vi "Test_CreateTable.vi"() -> ()   [LabVIEW 2020]
uses:
  C:/Program Files (x86)/National Instruments/LabVIEW 2018/vi.lib/Viviota/Viviota ORM/libraries/kdb/KpNet.KdbPlusClient.dll
  Program Files (x86)/National Instruments/LabVIEW 2018/vi.lib/Viviota/Viviota ORM/libraries/kdb/KpNet.KdbPlusClient.dll
  System.Data
  <vilib>/Viviota/VIV_Tools/Helpers.lvlib
panel:
  out "error out 3":errorcluster
  out "Array 7":string[](array[string])
  out "Array 6":variant[](array[variant])
  out "error out 2":errorcluster
  out "FieldCount 2":i32
  out "variant 4":variant
  out "variant 3":variant
  out "Array 5":string[](array[string])
  out "Array 4":variant[](array[variant])
  out "variant":variant
  out "GetName":string
  out "FieldCount":i32
  out "error out":errorcluster
  out "Array 3":string[](array[string])
  out "Array 2":variant[](array[variant])
  out "Read":bool
  out "Array":string[](array[string])
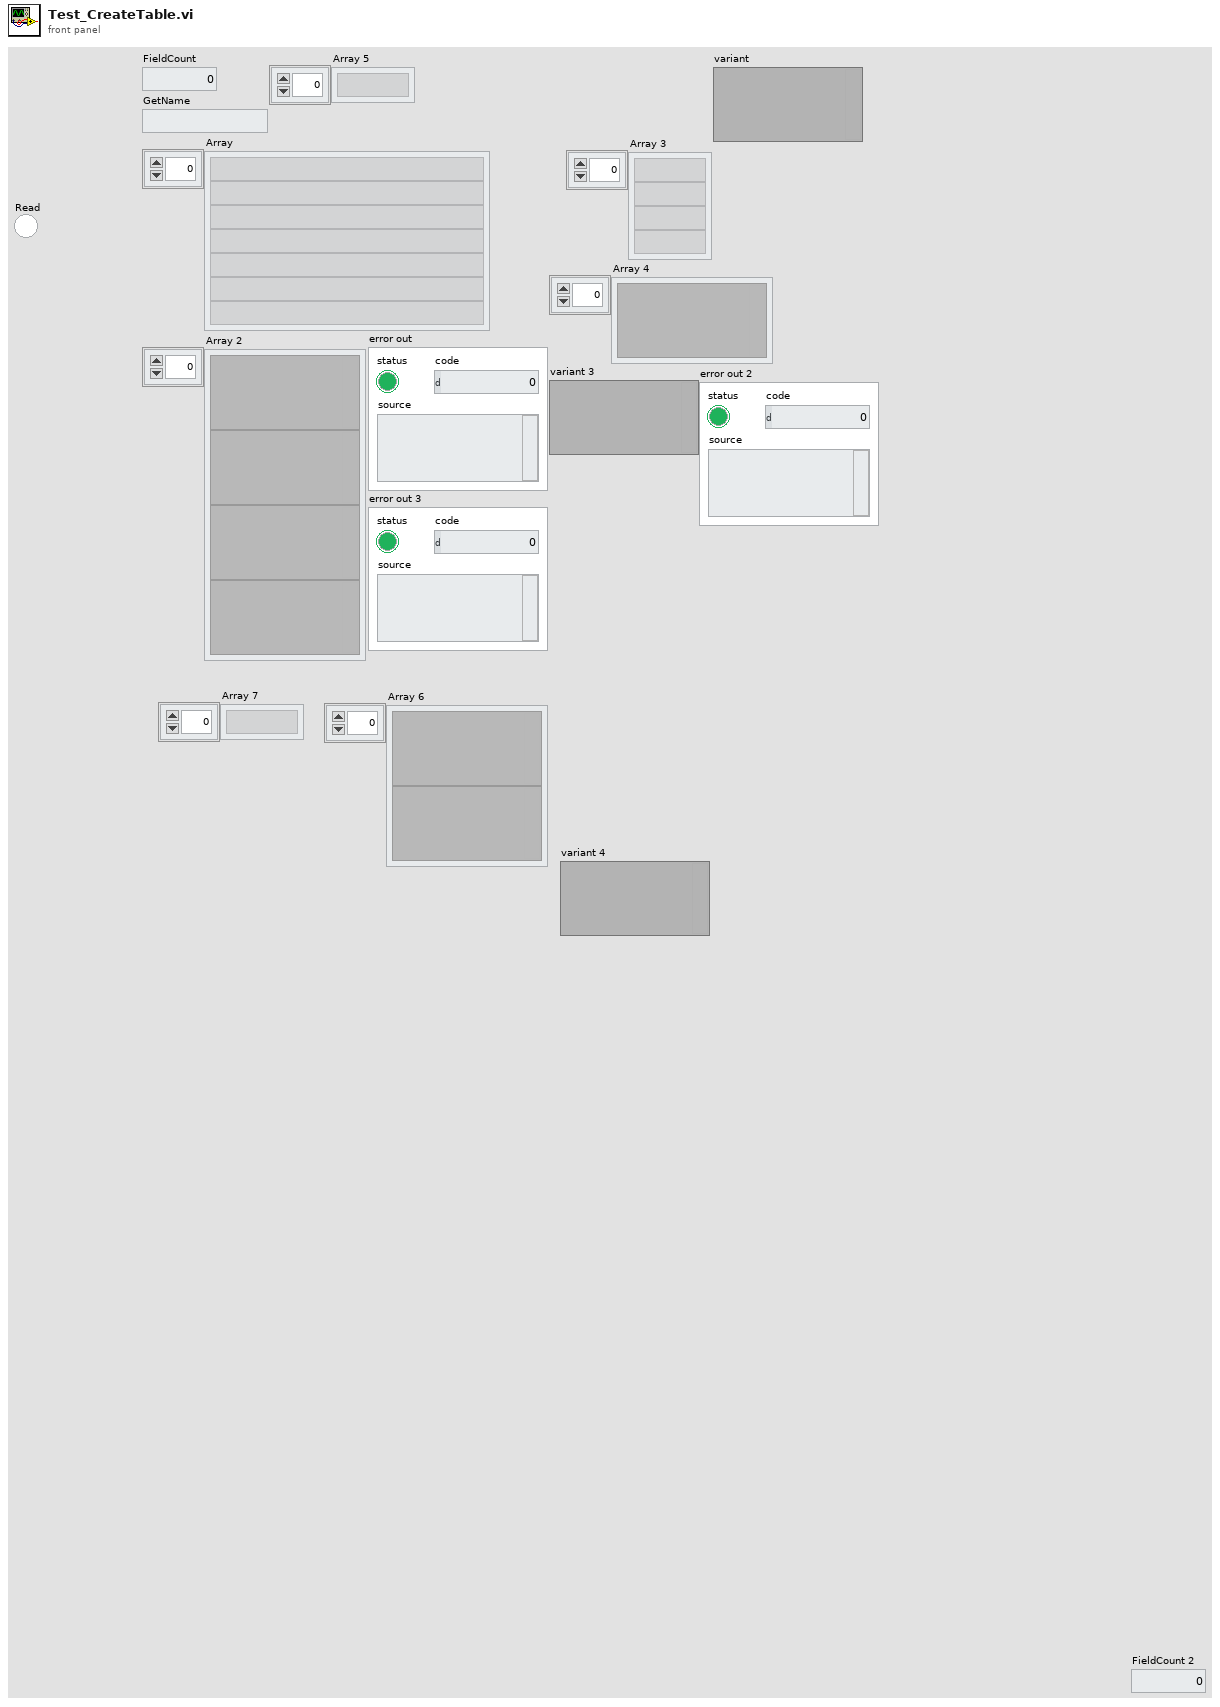
[diagram p1: front panel]
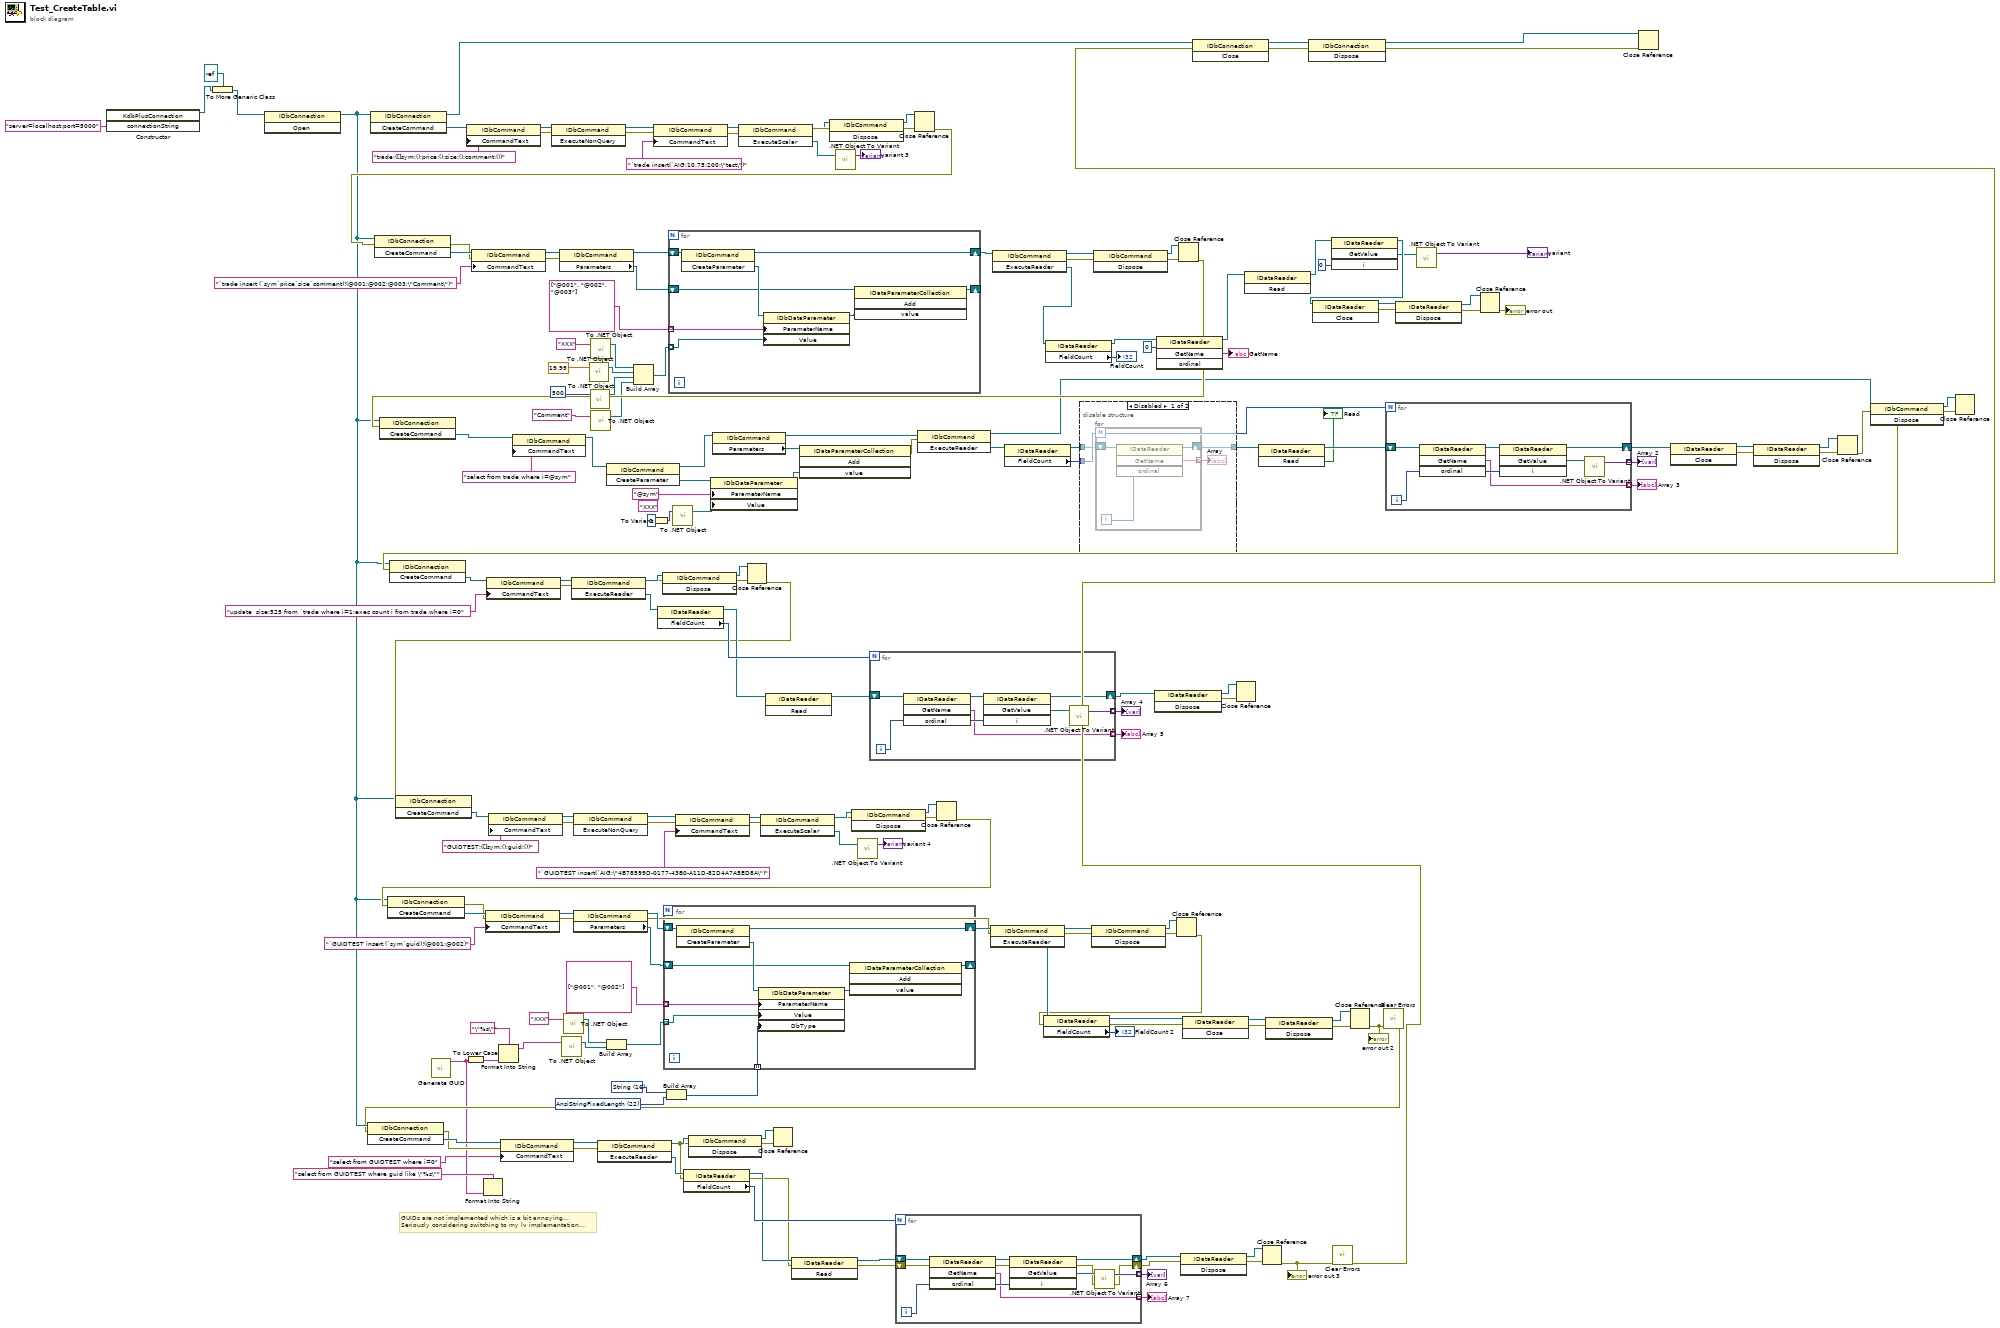
[diagram p0: block diagram]
diagram:
  w32 = 22 items=["AnsiString"=0, "Binary"=1, "Byte"=2, "Boolean"=3, "Currency"=4, "Date"=5, "DateTime"=6, "Decimal"=7, "Double"=8, "Guid"=9, "Int16"=10, "Int32"=11, "Int64"=12, "Object"=13, "SByte"=14, "Single"=15, "String"=16, "Time"=17, "UInt16"=18, "UInt32"=19, "UInt64"=20, "VarNumeric"=21, "AnsiStringFixedLength"=22, "StringFixedLength"=23, "Xml"=25, "DateTime2"=26, "DateTimeOffset"=27] ("DbType")
  w33 = 16 items=["AnsiString"=0, "Binary"=1, "Byte"=2, "Boolean"=3, "Currency"=4, "Date"=5, "DateTime"=6, "Decimal"=7, "Double"=8, "Guid"=9, "Int16"=10, "Int32"=11, "Int64"=12, "Object"=13, "SByte"=14, "Single"=15, "String"=16, "Time"=17, "UInt16"=18, "UInt32"=19, "UInt64"=20, "VarNumeric"=21, "AnsiStringFixedLength"=22, "StringFixedLength"=23, "Xml"=25, "DateTime2"=26, "DateTimeOffset"=27] ("DbType")
  (unwired) "XXX"
  # "GUIDs are not implemented which is a bit annoying...\nSeriously considering switching to my lv implementation..."
  n1 = constructor class="KdbPlusConnection"("connectionString"="server=localhost;port=5000") -> (reference out=w123:refnum<k24>)  [unwired: 3 in, 3 out]
  n2 = To More Generic Class(target class=refnum<k24> refnum ("connection"), reference=w123) -> (generic class reference=w122:refnum<k24>)
  n3 = invoke class="IDbConnection" method="Open"(reference=w122) -> (reference out=w25:refnum<k24>)  [unwired: 2 in, 2 out]
  n4 = invoke class="IDbConnection" method="CreateCommand"(reference=w25) -> (reference out=w125:refnum<k24>, "CreateCommand"=w189:refnum<k24>)  [unwired: 2 in, 1 out]
  n5 = call <vilib>:"Generate GUID.vi"() -> ("GUID"=w2:string)  [unwired: 9 in, 2 out]
  n6 = To Lower Case(string=w2) -> (all lower case string=w26:string)
  n7 = property class="IDbCommand"(reference=w189, "CommandText"="trade:([]sym:();price:();size:();comment:())") -> (reference out=w187:refnum<k24>, error out=w172:errorcluster)  [unwired: 1 in]
  n8 = Format Into String(format string="select from GUIDTEST where guid like \"%s\"" ("CommandText"), w2) -> ()  [unwired: 2 in, 2 out]
  n9 = Format Into String(format string="\"%s\"", w26) -> (resulting string=w30:string)  [unwired: 2 in, 1 out]
  n10 = invoke class="IDbCommand" method="ExecuteNonQuery"(reference=w187, error in=w172) -> (reference out=w174:refnum<k24>, error out=w173:errorcluster)  [unwired: 1 in, 1 out]
  n11 = call <vilib>:"To .NET Object.vi"("anything"=w30) -> (".NET object"=w52:refnum<k24>)  [unwired: 1 in, 1 out]
  n12 = call <vilib>:"To .NET Object.vi"("anything"="XXX") -> (".NET object"=w53:refnum<k24>)  [unwired: 1 in, 1 out]
  n13 = call <vilib>:"To .NET Object.vi"("anything"=19.99) -> (".NET object"=w146:refnum<k24>)  [unwired: 1 in, 1 out]
  n14 = call <vilib>:"To .NET Object.vi"("anything"=500) -> (".NET object"=w145:refnum<k24>)  [unwired: 1 in, 1 out]
  n15 = call <vilib>:"To .NET Object.vi"("anything"="XXX") -> (".NET object"=w147:refnum<k24>)  [unwired: 1 in, 1 out]
  n16 = call <vilib>:"To .NET Object.vi"("anything"="Comment") -> (".NET object"=w79:refnum<k24>)  [unwired: 1 in, 1 out]
  n17 = Build Array(w53, w52) -> (w51:refnum<k24>[])
  n18 = Build Array(w147, w146, w145, w79) -> (w144:refnum<k24>[])
  n19 = To Variant(anything=0) -> (Variant=w101:variant)
  n20 = property class="IDbCommand"(reference=w174, error in=w173, "CommandText"="`trade insert(`AIG;10.75;200;\"test\")") -> (reference out=w175:refnum<k24>, error out=w170:errorcluster)
  n21 = Build Array(w33, w32) -> (w31:i32[])
  n22 = call <vilib>:"To .NET Object.vi"("anything"=w101) -> (".NET object"=w162:refnum<k24>)  [unwired: 1 in, 1 out]
  n23 = invoke class="IDbCommand" method="ExecuteScalar"(reference=w175, error in=w170) -> (reference out=w140:refnum<k24>, error out=w141:errorcluster, "ExecuteScalar"=w82:refnum<k24>)  [unwired: 1 in]
  n24 = invoke class="IDbCommand" method="Dispose"(reference=w140, error in=w141) -> (reference out=w143:refnum<k24>, error out=w142:errorcluster)  [unwired: 1 in, 1 out]
  n25 = call <vilib>:".NET Object To Variant.vi"(".NET object"=w82) -> ("variant"=→"variant 3":variant)  [unwired: 1 in, 1 out]
  n26 = Close Reference(reference=w143, error in (no error)=w142) -> (error out=w132:errorcluster)
  n27 = invoke class="IDbConnection" method="CreateCommand"(reference=w25, error in=w132) -> (error out=w134:errorcluster, "CreateCommand"=w139:refnum<k24>)  [unwired: 1 in, 1 out]
  n28 = property class="IDbCommand"(reference=w139, error in=w134, "CommandText"="`trade insert (`sym`price`size`comment)!(@001;@002;@003;\"Comment\")") -> (reference out=w154:refnum<k24>, error out=w133:errorcluster)
  n29 = property class="IDbCommand"(reference=w154, error in=w133) -> (reference out=w153:refnum<k24>, "Parameters"=w152:refnum<k24>)  [unwired: 1 out]
  n30 = for {
    tunnel: w144 -> [w198] mode=indexing
    shift-right: [w194] -> _
    shift-left: w152 -> [w195]
    shift-right: [w193] -> w151
    shift-left: w153 -> [w196]
    tunnel: string[] ["@001", "@002", "@003"] -> [w192] mode=indexing
    n31 = invoke class="IDbCommand" method="CreateParameter"(reference=w196) -> (reference out=w193:refnum<k24>, "CreateParameter"=w197:refnum<k24>)  [unwired: 2 in, 1 out]
    n32 = property class="IDbDataParameter"(reference=w197, "ParameterName"=w192, "Value"=w198) -> (reference out=w191:refnum<k24>)  [unwired: 1 in, 1 out]
    n33 = invoke class="IDataParameterCollection" method="Add"(reference=w195, "value"=w191) -> (reference out=w194:refnum<k24>)  [unwired: 2 in, 3 out]
  }
  n34 = invoke class="IDbCommand" method="ExecuteReader"(reference=w151) -> (reference out=w136:refnum<k24>, error out=w135:errorcluster, "ExecuteReader"=w113:refnum<k24>)  [unwired: 2 in]
  n35 = property class="IDataReader"(reference=w113) -> (reference out=w111:refnum<k24>, "FieldCount"=→"FieldCount":i32)  [unwired: 1 in, 1 out]
  n36 = invoke class="IDbCommand" method="Dispose"(reference=w136, error in=w135) -> (reference out=w137:refnum<k24>, error out=w138:errorcluster)  [unwired: 1 in, 1 out]
  n37 = invoke class="IDataReader" method="GetName"(reference=w111, "ordinal"=0 ("i")) -> (reference out=w108:refnum<k24>, "GetName"=→"GetName":string)  [unwired: 2 in, 2 out]
  n38 = Close Reference(reference=w137, error in (no error)=w138) -> (error out=w130:errorcluster)
  n39 = invoke class="IDbConnection" method="CreateCommand"(reference=w25, error in=w130) -> ("CreateCommand"=w131:refnum<k24>)  [unwired: 1 in, 2 out]
  n40 = property class="IDbCommand"(reference=w131, "CommandText"="select from trade where i=@sym") -> (reference out=w176:refnum<k24>)  [unwired: 1 in, 1 out]
  n41 = invoke class="IDbCommand" method="CreateParameter"(reference=w176) -> (reference out=w177:refnum<k24>, "CreateParameter"=w181:refnum<k24>)  [unwired: 2 in, 1 out]
  n42 = property class="IDbDataParameter"(reference=w181, "ParameterName"="@sym", "Value"=w162) -> (reference out=w180:refnum<k24>)  [unwired: 1 in, 1 out]
  n43 = property class="IDbCommand"(reference=w177) -> (reference out=w178:refnum<k24>, "Parameters"=w182:refnum<k24>)  [unwired: 1 in, 1 out]
  n44 = invoke class="IDataParameterCollection" method="Add"(reference=w182, "value"=w180) -> (error out=w169:errorcluster)  [unwired: 2 in, 3 out]
  n45 = invoke class="IDbCommand" method="ExecuteReader"(reference=w178, error in=w169) -> (reference out=w126:refnum<k24>, "ExecuteReader"=w164:refnum<k24>)  [unwired: 1 in, 1 out]
  n46 = property class="IDataReader"(reference=w164) -> (reference out=w161:refnum<k24>, "FieldCount"=w120:i32)  [unwired: 1 in, 1 out]
  n47 = disable-structure shown="Disabled" {
    disable-tunnel: w161 -> [w201 w207]
    disable-tunnel: [w200 w207] -> w160
    disable-tunnel: w120 -> [w199 _]
    frame Disabled {
      n48 = for {
        N: w199 -> [_]
        tunnel: [w205] -> w202 mode=indexing
        shift-right: [w206] -> w200
        shift-left: w201 -> [w204]
        i -> [w203]
        n49 = invoke class="IDataReader" method="GetName"(reference=w204, "ordinal"=w203) -> (reference out=w206:refnum<k24>, "GetName"=w205:string)  [unwired: 2 in, 2 out]
      }
      "Array" <- w202
    }
    frame Enabled {
    }
  }
  n50 = invoke class="IDataReader" method="Read"(reference=w108) -> (reference out=w107:refnum<k24>)  [unwired: 2 in, 2 out]
  n51 = invoke class="IDataReader" method="Read"(reference=w160) -> (reference out=w159:refnum<k24>, "Read"=→"Read":bool)  [unwired: 2 in, 1 out]
  n52 = invoke class="IDataReader" method="GetValue"(reference=w107, "i"=0) -> (reference out=w106:refnum<k24>, "GetValue"=w104:refnum<k24>)  [unwired: 2 in, 2 out]
  n53 = invoke class="IDataReader" method="Close"(reference=w106) -> (reference out=w115:refnum<k24>, error out=w116:errorcluster)  [unwired: 2 in, 1 out]
  n54 = for {
    N: w120 -> [_]
    shift-right: [w214] -> w158
    shift-left: w159 -> [w211]
    tunnel: [w212] -> w121 mode=indexing
    tunnel: [w208] -> w119 mode=indexing
    i -> [w209]
    n55 = invoke class="IDataReader" method="GetName"(reference=w211, "ordinal"=w209) -> (reference out=w210:refnum<k24>, "GetName"=w208:string)  [unwired: 2 in, 2 out]
    n56 = invoke class="IDataReader" method="GetValue"(reference=w210, "i"=w209) -> (reference out=w214:refnum<k24>, "GetValue"=w213:refnum<k24>)  [unwired: 2 in, 2 out]
    n57 = call <vilib>:".NET Object To Variant.vi"(".NET object"=w213) -> ("variant"=w212:variant)  [unwired: 1 in, 1 out]
  }
  "Array 2" <- w121
  "Array 3" <- w119
  n58 = invoke class="IDataReader" method="Dispose"(reference=w115, error in=w116) -> (reference out=w118:refnum<k24>, error out=w117:errorcluster)  [unwired: 1 in, 1 out]
  n59 = call <vilib>:".NET Object To Variant.vi"(".NET object"=w104) -> ("variant"=→"variant":variant)  [unwired: 1 in, 1 out]
  n60 = Close Reference(reference=w118, error in (no error)=w117) -> (error out=→"error out":errorcluster)
  n61 = invoke class="IDataReader" method="Close"(reference=w158) -> (reference out=w168:refnum<k24>, error out=w167:errorcluster)  [unwired: 2 in, 1 out]
  n62 = invoke class="IDataReader" method="Dispose"(reference=w168, error in=w167) -> (reference out=w165:refnum<k24>, error out=w166:errorcluster)  [unwired: 1 in, 1 out]
  n63 = Close Reference(reference=w165, error in (no error)=w166) -> (error out=w127:errorcluster)
  n64 = invoke class="IDbCommand" method="Dispose"(reference=w126, error in=w127) -> (reference out=w128:refnum<k24>, error out=w129:errorcluster)  [unwired: 1 in, 1 out]
  n65 = Close Reference(reference=w128, error in (no error)=w129) -> (error out=w92:errorcluster)
  n66 = invoke class="IDbConnection" method="CreateCommand"(reference=w25, error in=w92) -> ("CreateCommand"=w93:refnum<k24>)  [unwired: 1 in, 2 out]
  n67 = property class="IDbCommand"(reference=w93, "CommandText"="update  size:525 from `trade where i=1;exec count i from trade where i=0") -> (reference out=w94:refnum<k24>, error out=w96:errorcluster)  [unwired: 1 in]
  n68 = invoke class="IDbCommand" method="ExecuteReader"(reference=w94, error in=w96) -> (reference out=w100:refnum<k24>, error out=w99:errorcluster, "ExecuteReader"=w91:refnum<k24>)  [unwired: 1 in]
  n69 = property class="IDataReader"(reference=w91) -> (reference out=w84:refnum<k24>, "FieldCount"=w88:i32)  [unwired: 1 in, 1 out]
  n70 = invoke class="IDbCommand" method="Dispose"(reference=w100, error in=w99) -> (reference out=w97:refnum<k24>, error out=w98:errorcluster)  [unwired: 1 in, 1 out]
  n71 = Close Reference(reference=w97, error in (no error)=w98) -> (error out=w63:errorcluster)
  n72 = invoke class="IDbConnection" method="CreateCommand"(reference=w25, error in=w63) -> ("CreateCommand"=w64:refnum<k24>)  [unwired: 1 in, 2 out]
  n73 = property class="IDbCommand"(reference=w64, "CommandText"="GUIDTEST:([]sym:();guid:())") -> (reference out=w66:refnum<k24>, error out=w70:errorcluster)  [unwired: 1 in]
  n74 = invoke class="IDbCommand" method="ExecuteNonQuery"(reference=w66, error in=w70) -> (reference out=w68:refnum<k24>, error out=w69:errorcluster)  [unwired: 1 in, 1 out]
  n75 = property class="IDbCommand"(reference=w68, error in=w69, "CommandText"="`GUIDTEST insert(`AIG;\"4B78599D-0177-43B0-A11D-82D4A7A5ED8A\")") -> (reference out=w67:refnum<k24>, error out=w72:errorcluster)
  n76 = invoke class="IDbCommand" method="ExecuteScalar"(reference=w67, error in=w72) -> (reference out=w76:refnum<k24>, error out=w75:errorcluster, "ExecuteScalar"=w77:refnum<k24>)  [unwired: 1 in]
  n77 = invoke class="IDataReader" method="Read"(reference=w84) -> (reference out=w83:refnum<k24>)  [unwired: 2 in, 2 out]
  n78 = invoke class="IDbCommand" method="Dispose"(reference=w76, error in=w75) -> (reference out=w73:refnum<k24>, error out=w74:errorcluster)  [unwired: 1 in, 1 out]
  n79 = call <vilib>:".NET Object To Variant.vi"(".NET object"=w77) -> ("variant"=→"variant 4":variant)  [unwired: 1 in, 1 out]
  n80 = for {
    N: w88 -> [_]
    shift-right: [w221] -> w87
    shift-left: w83 -> [w218]
    tunnel: [w219] -> w86 mode=indexing
    tunnel: [w215] -> w85 mode=indexing
    i -> [w216]
    n81 = invoke class="IDataReader" method="GetName"(reference=w218, "ordinal"=w216) -> (reference out=w217:refnum<k24>, "GetName"=w215:string)  [unwired: 2 in, 2 out]
    n82 = invoke class="IDataReader" method="GetValue"(reference=w217, "i"=w216) -> (reference out=w221:refnum<k24>, "GetValue"=w220:refnum<k24>)  [unwired: 2 in, 2 out]
    n83 = call <vilib>:".NET Object To Variant.vi"(".NET object"=w220) -> ("variant"=w219:variant)  [unwired: 1 in, 1 out]
  }
  "Array 4" <- w86
  "Array 5" <- w85
  n84 = Close Reference(reference=w73, error in (no error)=w74) -> (error out=w35:errorcluster)
  n85 = invoke class="IDbConnection" method="CreateCommand"(reference=w25, error in=w35) -> (error out=w59:errorcluster, "CreateCommand"=w60:refnum<k24>)  [unwired: 1 in, 1 out]
  n86 = property class="IDbCommand"(reference=w60, error in=w59, "CommandText"="`GUIDTEST insert (`sym`guid)!(@001;@002)") -> (reference out=w61:refnum<k24>, error out=w58:errorcluster)
  n87 = property class="IDbCommand"(reference=w61, error in=w58) -> (reference out=w56:refnum<k24>, error out=w44:errorcluster, "Parameters"=w57:refnum<k24>)
  n88 = for {
    tunnel: w51 -> [w230] mode=indexing
    shift-right: [w226] -> _
    shift-left: w57 -> [w227]
    shift-right: [w225] -> w45
    shift-left: w56 -> [w228]
    tunnel: string[] ["@001", "@002"] -> [w224] mode=indexing
    tunnel: w31 -> [w222] mode=indexing
    n89 = invoke class="IDbCommand" method="CreateParameter"(reference=w228) -> (reference out=w225:refnum<k24>, "CreateParameter"=w229:refnum<k24>)  [unwired: 2 in, 1 out]
    n90 = property class="IDbDataParameter"(reference=w229, "ParameterName"=w224, "Value"=w230, "DbType"=w222) -> (reference out=w223:refnum<k24>)  [unwired: 1 in, 1 out]
    n91 = invoke class="IDataParameterCollection" method="Add"(reference=w227, "value"=w223) -> (reference out=w226:refnum<k24>)  [unwired: 2 in, 3 out]
  }
  n92 = invoke class="IDbCommand" method="ExecuteReader"(reference=w45, error in=w44) -> (reference out=w48:refnum<k24>, error out=w47:errorcluster, "ExecuteReader"=w43:refnum<k24>)  [unwired: 1 in]
  n93 = invoke class="IDbCommand" method="Dispose"(reference=w48, error in=w47) -> (reference out=w49:refnum<k24>, error out=w50:errorcluster)  [unwired: 1 in, 1 out]
  n94 = invoke class="IDataReader" method="Dispose"(reference=w87) -> (reference out=w90:refnum<k24>, error out=w89:errorcluster)  [unwired: 2 in, 1 out]
  n95 = Close Reference(reference=w49, error in (no error)=w50) -> (error out=w36:errorcluster)
  n96 = property class="IDataReader"(reference=w43, error in=w36) -> (reference out=w38:refnum<k24>, error out=w37:errorcluster, "FieldCount"=→"FieldCount 2":i32)
  n97 = invoke class="IDataReader" method="Close"(reference=w38, error in=w37) -> (reference out=w42:refnum<k24>, error out=w41:errorcluster)  [unwired: 1 in, 1 out]
  n98 = Close Reference(reference=w90, error in (no error)=w89) -> ()  [unwired: 1 out]
  n99 = invoke class="IDataReader" method="Dispose"(reference=w42, error in=w41) -> (reference out=w39:refnum<k24>, error out=w40:errorcluster)  [unwired: 1 in, 1 out]
  n100 = Close Reference(reference=w39, error in (no error)=w40) -> (error out=w34:errorcluster)
  "error out 2" <- w34
  n101 = call <vilib>:"Clear Errors.vi"("error in (no error)"=w34) -> ("error out"=w3:errorcluster)  [unwired: 5 in, 1 out]
  n102 = invoke class="IDbConnection" method="CreateCommand"(reference=w25, error in=w3) -> (error out=w11:errorcluster, "CreateCommand"=w28:refnum<k24>)  [unwired: 1 in, 1 out]
  n103 = property class="IDbCommand"(reference=w28, error in=w11, "CommandText"="select from GUIDTEST where i=0") -> (reference out=w12:refnum<k24>, error out=w10:errorcluster)
  n104 = invoke class="IDbCommand" method="ExecuteReader"(reference=w12, error in=w10) -> (reference out=w24:refnum<k24>, error out=w9:errorcluster, "ExecuteReader"=w21:refnum<k24>)  [unwired: 1 in]
  n105 = property class="IDataReader"(reference=w21, error in=w9) -> (reference out=w14:refnum<k24>, error out=w8:errorcluster, "FieldCount"=w18:i32)
  n106 = invoke class="IDbCommand" method="Dispose"(reference=w24, error in=w9) -> (reference out=w22:refnum<k24>, error out=w23:errorcluster)  [unwired: 1 in, 1 out]
  n107 = Close Reference(reference=w22, error in (no error)=w23) -> ()  [unwired: 1 out]
  n108 = invoke class="IDataReader" method="Read"(reference=w14, error in=w8) -> (reference out=w13:refnum<k24>, error out=w6:errorcluster)  [unwired: 1 in, 1 out]
  n109 = for {
    N: w18 -> [_]
    shift-right: [w241] -> w17
    shift-left: w13 -> [w238]
    tunnel: [w239] -> w16 mode=indexing
    tunnel: [w235] -> w15 mode=indexing
    shift-right: [w232] -> w5
    shift-left: w6 -> [w234]
    i -> [w236]
    n110 = invoke class="IDataReader" method="GetName"(reference=w238, error in=w234, "ordinal"=w236) -> (reference out=w237:refnum<k24>, error out=w231:errorcluster, "GetName"=w235:string)  [unwired: 1 in, 1 out]
    n111 = invoke class="IDataReader" method="GetValue"(reference=w237, error in=w231, "i"=w236) -> (reference out=w241:refnum<k24>, error out=w233:errorcluster, "GetValue"=w240:refnum<k24>)  [unwired: 1 in, 1 out]
    n112 = call <vilib>:".NET Object To Variant.vi"("error in (no error)"=w233, ".NET object"=w240) -> ("error out"=w232:errorcluster, "variant"=w239:variant)
  }
  "Array 6" <- w16
  "Array 7" <- w15
  n113 = invoke class="IDataReader" method="Dispose"(reference=w17, error in=w5) -> (reference out=w20:refnum<k24>, error out=w19:errorcluster)  [unwired: 1 in, 1 out]
  n114 = Close Reference(reference=w20, error in (no error)=w19) -> (error out=w7:errorcluster)
  "error out 3" <- w7
  n115 = call <vilib>:"Clear Errors.vi"("error in (no error)"=w7) -> ("error out"=w4:errorcluster)  [unwired: 5 in, 1 out]
  n116 = invoke class="IDbConnection" method="Close"(reference=w125, error in=w4) -> (reference out=w186:refnum<k24>, error out=w183:errorcluster)  [unwired: 1 in, 1 out]
  n117 = invoke class="IDbConnection" method="Dispose"(reference=w186, error in=w183) -> (reference out=w184:refnum<k24>, error out=w185:errorcluster)  [unwired: 1 in, 1 out]
  n118 = Close Reference(reference=w184, error in (no error)=w185) -> ()  [unwired: 1 out]
